vi "Get Key.vi"(8 "error in (no error)":errorcluster, 11 "Attribute in":refnum<class "Attribute.lvclass">) -> (0 "error out":errorcluster, 2 "Key":string, 3 "Attribute out":refnum<class "Attribute.lvclass">)   [LabVIEW 2019, in "HierDAL Library.lvlib" / "Models.lvlib" / "Attribute.lvclass"]
uses:
  Attribute.lvclass
  Attribute.lvclass/Attribute.ctl
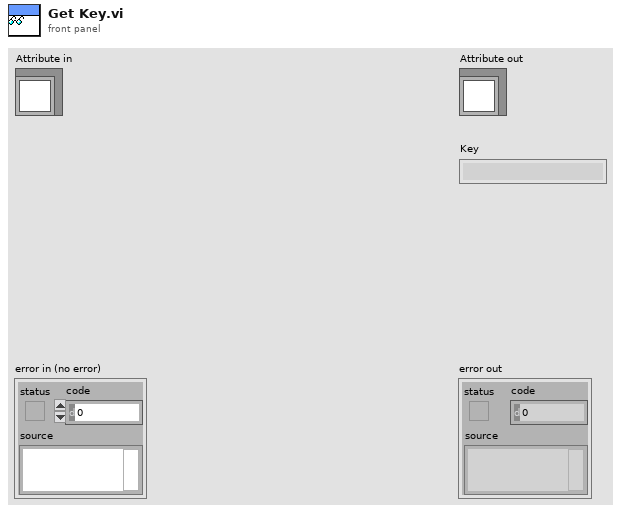
[diagram p1: front panel]
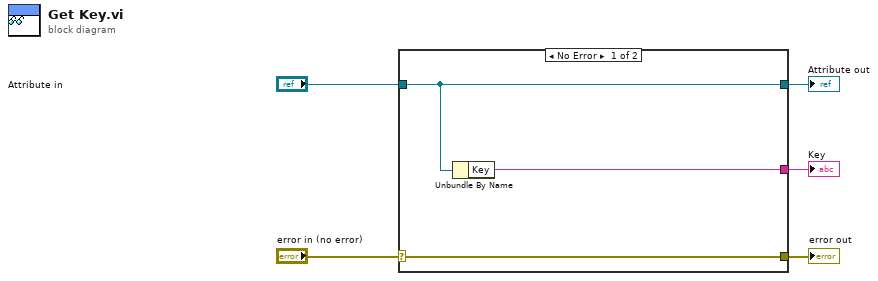
[diagram p0: block diagram]
diagram:
  n1 = case shown="No Error" "error in (no error)" {
    selector: "error in (no error)" -> [w8 w9]
    tunnel: [w8 w9] -> w4
    tunnel: [w7 w10] -> w2
    tunnel: "Attribute in" -> [w7 w10]
    tunnel: [w6 _] -> w1
    frame No Error {
      n2 = Unbundle By Name(w7) -> ("Key"=w6:string)
    }
    frame Error {
    }
  }
  "error out" <- w4
  "Attribute out" <- w2
  "Key" <- w1
